vi "Array Control Constant Indicator.vi"() -> ()   [LabVIEW 2015]
panel:
  out "size(s) 3":i32[](array[numeric])
  in  "String 2D Array  2":string[][](array[string])
  out "String 2D Array Indicator 3":string[][](array[string])
  out "Numeric 1D Array Indicator 2":string[](array[string])
  in  "String 1D Array":string[](array[string])
  out "Numeric 1D Array Indicator":dbl[](array[slide]) scale=0.0..10.0
  in  "Numeric 1D Array":dbl[](array[slide]) scale=0.0..10.0
  out "size(s) 2":i32
  out "Boelaen 1D Array Indicator 2":bool[](array[boolean])
  out "Boelaen 1D Array Indicator":bool[](array[boolean])
  out "size(s)":i32
  in  "Boelaen 1D Array":bool[](array[boolean])
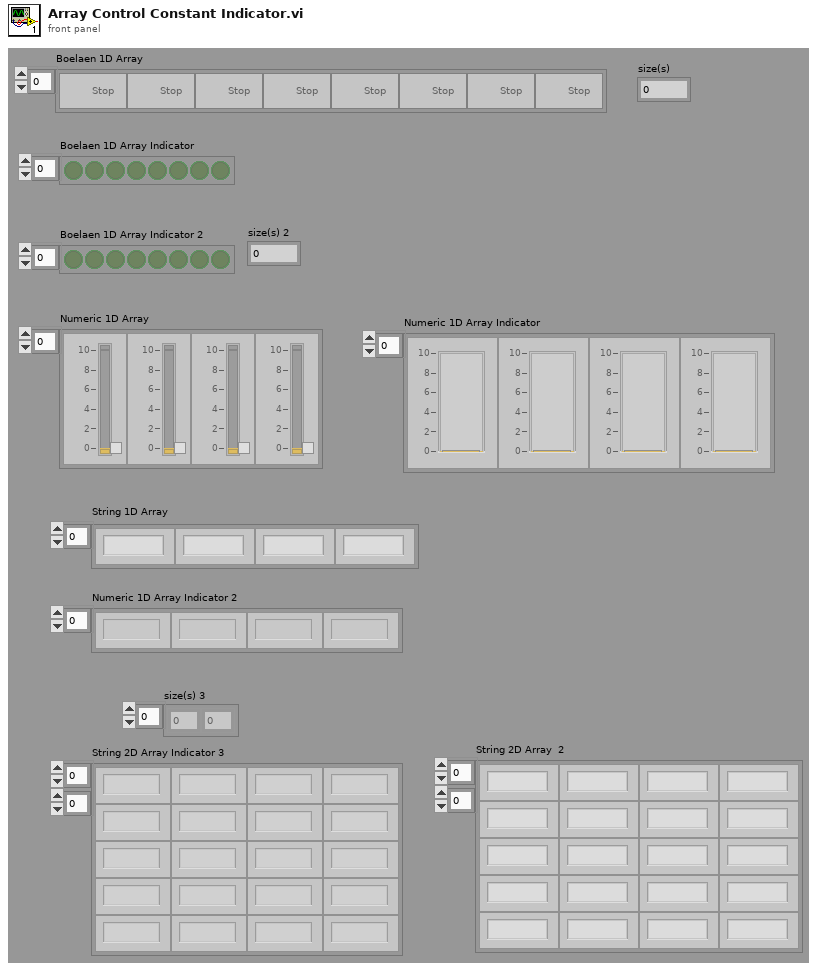
[diagram p1: front panel]
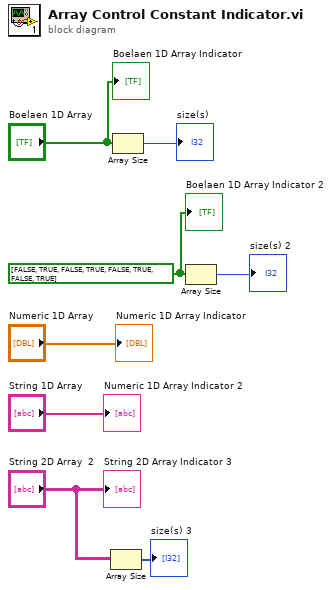
[diagram p0: block diagram]
diagram:
  w5 = bool[] [FALSE, TRUE, FALSE, TRUE, FALSE, TRUE, FALSE, TRUE] ("Boelaen 1D Array 2")
  n1 = Array Size(array="String 2D Array  2") -> (size(s)=→"size(s) 3":i32[])
  n2 = Array Size(array="Boelaen 1D Array") -> (size(s)=→"size(s)":i32)
  n3 = Array Size(array=w5) -> (size(s)=→"size(s) 2":i32)
  "Boelaen 1D Array Indicator" <- "Boelaen 1D Array"
  "Boelaen 1D Array Indicator 2" <- w5
  "Numeric 1D Array Indicator" <- "Numeric 1D Array"
  "Numeric 1D Array Indicator 2" <- "String 1D Array"
  "String 2D Array Indicator 3" <- "String 2D Array  2"
